vi "1500_DAQ.vi"(8 "error in":errorcluster) -> (0 "error out":errorcluster, 1 "输入":waveform(dbl)(graph), 2 "方波刺激":waveform(dbl)(graph), 3 "电阻值 2":dbl)   [LabVIEW 2016]
uses:
  <vilib>/DAQmx/write.llb/DAQmx Write (Analog Wfm 1Chan NSamp).vi
  <vilib>/DAQmx/read.llb/DAQmx Read (Analog Wfm 1Chan NSamp).vi
  <vilib>/Analysis/baseanly.llb/Mean (DBL).vi
  <vilib>/Waveform/WDTOps.llb/WDT Waveform Duration DBL.vi
  <vilib>/DAQmx/create/channels.llb/DAQmx Create Channel (AI-Voltage-Basic).vi
  <vilib>/DAQmx/configure/timing.llb/DAQmx Timing (Sample Clock).vi
  <vilib>/DAQmx/create/channels.llb/DAQmx Create Channel (AO-Voltage-Basic).vi
  <vilib>/DAQmx/miscellaneous.llb/DAQmx Fill In Error Info.vi
  <vilib>/measure/NI_MABase.lvlib
  <resource>/objmgr/daqmx.rc
  <vilib>/Analysis/NI_AALBase.lvlib
panel:
  out "阻值波形图表":dbl(graph)
  out "Resistance":dbl
  out "Negative Peak":dbl
  out "前半段波形图":dbl[](graph)
  out "后半段波形图 2":dbl[](graph)
  out "最小值":dbl
  out "mean":dbl caption="均值" format="%0.2f"
  in  "Holding Voltage":dbl
  in  "amplitude":dbl=0.02
  in  "Averaging":i32=7
  in  "frequency":dbl=20.0
  in  "下拉列表":u16(ring)=1 items=["Current Clamp", "Voltage Clamp"]
  out "Waveform Graph":waveform(dbl)[](graph)
  in  "Initialize?":bool
  out "实际采样率":dbl=1000.0 format="%0.2f"
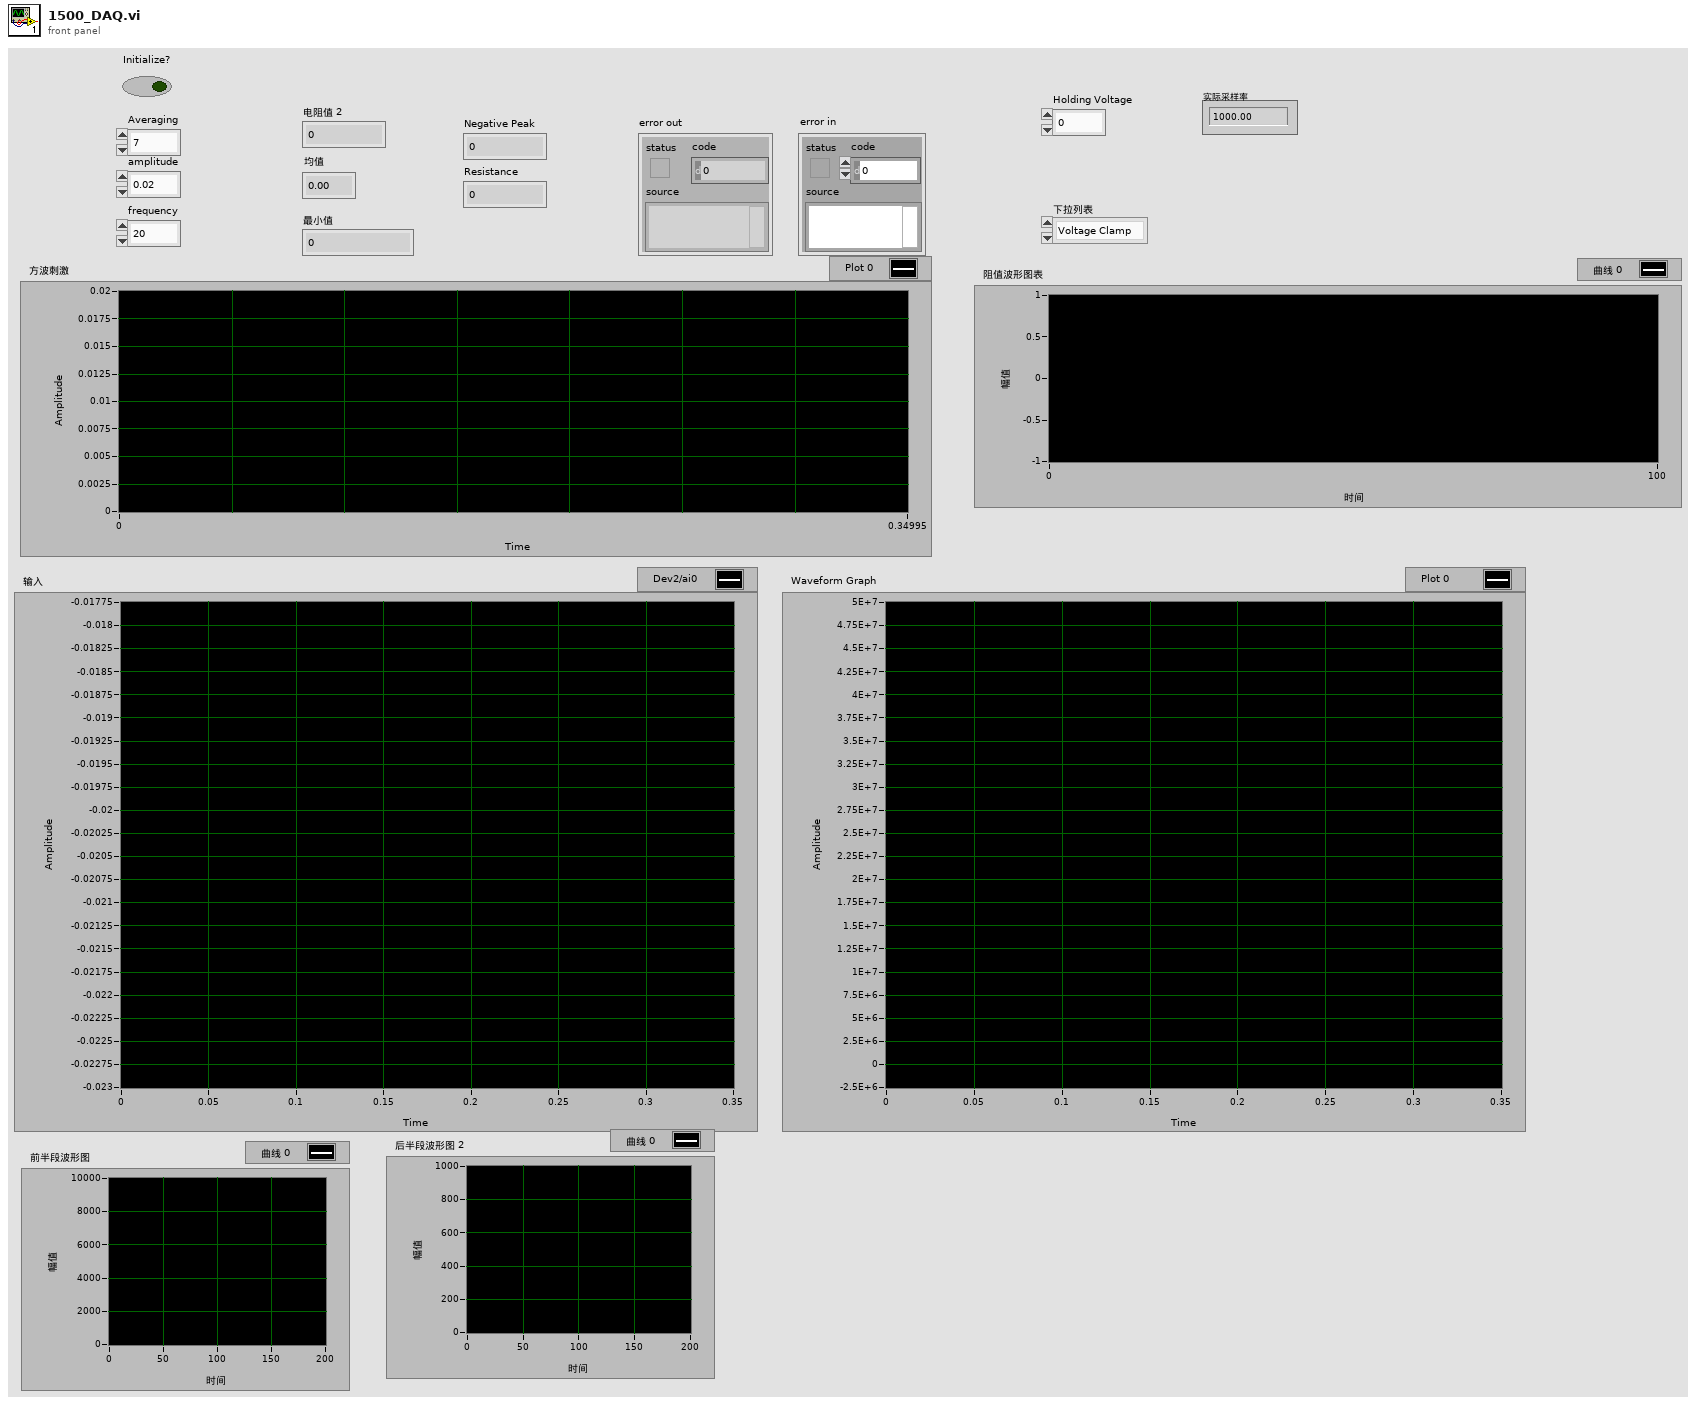
[diagram p1: front panel]
types:
  T1 = enum16{"Sine Wave", "Triangle Wave", "Square Wave", "Sawtooth Wave"}
  T2 = cluster{"Averaging":i32, "frequency":dbl, "amplitude":dbl, "Proportion":dbl, "Fs":dbl}
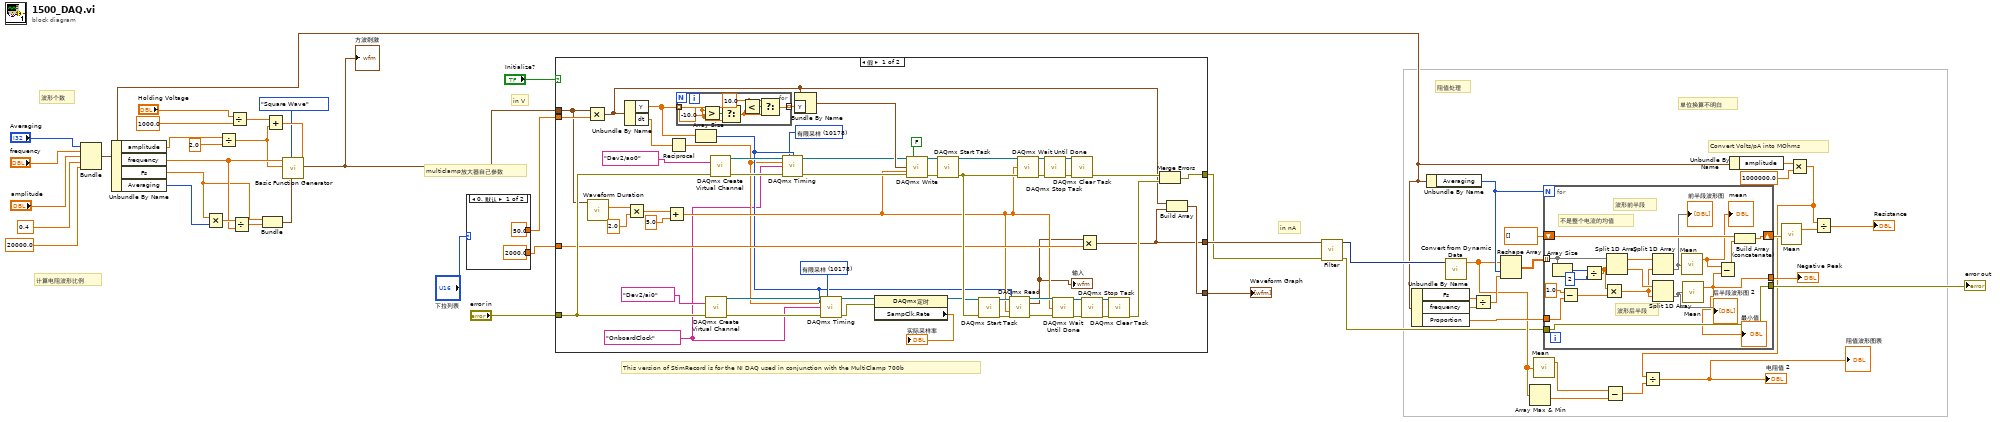
[diagram p0: block diagram]
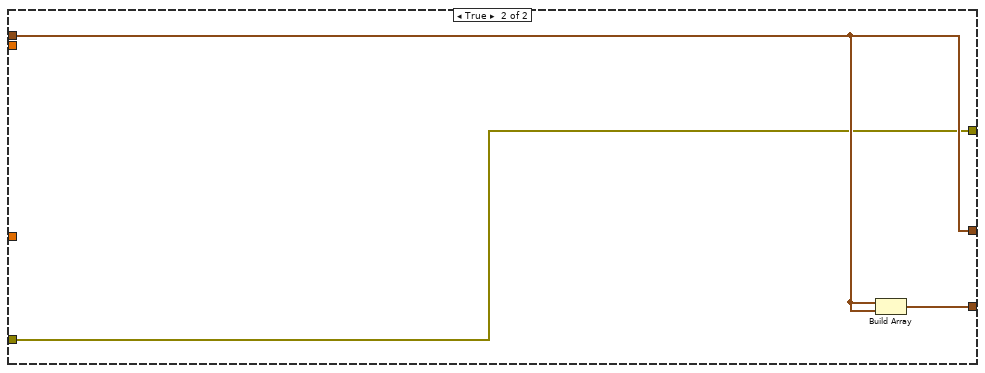
[diagram p2: hidden frame]
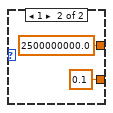
[diagram p3: hidden frame]
diagram:
  # "单位换算不明白"
  # "阻值处理"
  # "Convert Volts/pA into MOhms"
  # "波形个数"
  # "计算电阻波形比例"
  # "This version of StimRecord is for the NI DAQ used in conjunction with the MultiClamp 700b"
  # "multiclamp放大器自己参数"
  # "in V"
  # "in nA"
  n1 = Bundle("Averaging"="Averaging", "frequency"="frequency", "amplitude"="amplitude", "Proportion"=0.4, "Fs"=20000.0) -> (w1:T2)  [unwired: 1 in]
  n2 = Unbundle By Name(w1) -> ("amplitude"=w36:dbl, "frequency"=w37:dbl, "Fs"=w35:dbl, "Averaging"=w34:i32)
  n3 = Multiply(x=w35, y=w34) -> (x*y=w39:dbl)
  n4 = Divide(x=w36, y=2.0) -> (x/y=w31:dbl)
  n5 = Divide(x="Holding Voltage", y=1000.0) -> (x/y=w30:dbl)
  n6 = Divide(x=w39, y=w37) -> (x/y=w38:dbl)
  n7 = Bundle("Fs"=w35, w38) -> (w33:cluster{"Fs":dbl, dbl})  [unwired: 1 in]
  n8 = Add(x=w30, y=w31) -> (x+y=w32:dbl)
  n9 = call <vilib>:"Basic Function Generator.vi"("offset"=w32, "sampling info"=w33, "signal type"=T1."Square Wave", "amplitude"=w31, "frequency"=w37) -> ("signal out"=w26:waveform(dbl))  [unwired: 4 in, 2 out]
  "方波刺激" <- w26
  n10 = case shown="0, 默认" "下拉列表" {
    tunnel: [50.0 ("y") 2500000000.0 ("y")] -> w49
    tunnel: [2000.0 ("y") 0.1 ("y")] -> w48
    frame 0, Default {
    }
    frame 1 {
    }
  }
  n11 = case shown="假" "Initialize?" {
    tunnel: "error in" -> [w89 w117]
    tunnel: [w88 w117] -> w2
    tunnel: [w86 w119] -> w4
    tunnel: w26 -> [w75 w119]
    tunnel: [w87 w118] -> w50
    tunnel: w49 -> [w77 _]
    tunnel: w48 -> [w76 _]
    frame False {
      w57 = 10178 items=["有限采样"=10178, "连续采样"=10123, "硬件定时单点"=12522] ("sample mode")
      w56 = tag "OnboardClock" ("source")
      w66 = 10178 items=["有限采样"=10178, "连续采样"=10123, "硬件定时单点"=12522] ("sample mode")
      n12 = Multiply(x=w75, y=w77) -> (x*y=w84:waveform(dbl))
      n13 = call-poly <vilib>:"Waveform Duration.vi"("waveform in"=w75) -> ("duration"=w73:dbl)  [unwired: 8 in, 2 out]
      n14 = Unbundle By Name(w84) -> ("Y"=w79:dbl[], "dt"=w90:dbl)
      n15 = Multiply(x=w73, y=2.0) -> (x*y=w71:dbl)
      n16 = Add(x=w71, y=5.0) -> (x+y=w72:dbl)
      n17 = Reciprocal(x=w90) -> (1/x=w64:dbl)
      n18 = for {
        tunnel: [w116] -> w85 mode=indexing
        tunnel: w79 -> [w110] mode=indexing
        w111 = 10.0 ("t")
        w114 = -10.0 ("t")
        n19 = Greater?(x=w114, y=w110) -> (0:w115:bool)
        n20 = Select(t=w114, s=w115, f=w110) -> (s? t:f=w112:dbl)
        n21 = Less?(x=w111, y=w112) -> (x < y?=w113:bool)
        n22 = Select(t=w111, s=w113, f=w112) -> (s? t:f=w116:dbl)
      }
      n23 = Array Size(array=w79) -> (size(s)=w65:i32)
      n24 = call-poly <vilib>:"DAQmx Create Virtual Channel.vi"("physical channels"=tag "Dev2/ai0", "error in"=w89) -> ("task out"=w67:refnum<k21>, "error out"=w68:errorcluster)  [unwired: 12 in]
      n25 = call-poly <vilib>:"DAQmx Create Virtual Channel.vi"("physical channels"=tag "Dev2/ao0", "error in"=w89) -> ("task out"=w95:refnum<k21>, "error out"=w96:errorcluster)  [unwired: 12 in]
      n26 = call-poly <vilib>:"DAQmx Timing.vi"("task/channels in"=w95, "sample mode"=w57, "samples per channel"=w65, "rate"=w64, "source"=w56, "error in"=w96) -> ("task out"=w81:refnum<k21>, "error out"=w80:errorcluster)  [unwired: 8 in]
      n27 = Bundle By Name(cluster=w84, "Y"=w85) -> (w83:waveform(dbl))
      n28 = call-poly <vilib>:"DAQmx Timing.vi"("task/channels in"=w67, "sample mode"=w66, "samples per channel"=w65, "rate"=w64, "source"=w56, "error in"=w68) -> ("task out"=w62:refnum<k21>, "error out"=w61:errorcluster)  [unwired: 8 in]
      n29 = property class="DAQmx定时"(reference=w62, error in=w61) -> (reference out=w60:refnum<k21>, "SampClk.Rate"=→"实际采样率":dbl)  [unwired: 1 out]
      n30 = call-poly <vilib>:"DAQmx Write.vi"("task/channels in"=w81, "auto start"=FALSE, "data"=w83, "timeout"=w72, "error in"=w80) -> ("task out"=w91:refnum<k21>, "error out"=w82:errorcluster)  [unwired: 8 in, 1 out]
      n31 = call <vilib>:"DAQmx Start Task.vi"("task/channels in"=w91, "error in"=w82) -> ("task out"=w92:refnum<k21>, "error out"=w78:errorcluster)  [unwired: 12 in]
      n32 = call <vilib>:"DAQmx Start Task.vi"("task/channels in"=w60, "error in"=w78) -> ("task out"=w100:refnum<k21>, "error out"=w99:errorcluster)  [unwired: 12 in]
      n33 = call-poly <vilib>:"DAQmx Read.vi"("task/channels in"=w100, "number of samples per channel"=w65, "timeout"=w72, "error in"=w99) -> ("task out"=w106:refnum<k21>, "data"=w69:waveform(dbl), "error out"=w105:errorcluster)  [unwired: 9 in]
      "输入" <- w69
      n34 = call <vilib>:"DAQmx Wait Until Done.vi"("task/channels in"=w92, "timeout (sec)"=w72, "error in"=w78) -> ("task out"=w94:refnum<k21>, "error out"=w93:errorcluster)  [unwired: 11 in]
      n35 = call <vilib>:"DAQmx Stop Task.vi"("task/channels in"=w94, "error in"=w93) -> ("task out"=w97:refnum<k21>, "error out"=w98:errorcluster)  [unwired: 12 in]
      n36 = call <vilib>:"DAQmx Wait Until Done.vi"("task/channels in"=w106, "timeout (sec)"=w72, "error in"=w105) -> ("task out"=w104:refnum<k21>, "error out"=w103:errorcluster)  [unwired: 11 in]
      n37 = call <vilib>:"DAQmx Clear Task.vi"("task in"=w97, "error in"=w98) -> ("error out"=w108:errorcluster)  [unwired: 13 in]
      n38 = Multiply(x=w69, y=w76) -> (x*y=w86:waveform(dbl))
      n39 = call <vilib>:"DAQmx Stop Task.vi"("task/channels in"=w104, "error in"=w103) -> ("task out"=w102:refnum<k21>, "error out"=w101:errorcluster)  [unwired: 12 in]
      n40 = call <vilib>:"DAQmx Clear Task.vi"("task in"=w102, "error in"=w101) -> ("error out"=w107:errorcluster)  [unwired: 13 in]
      n41 = Merge Errors(w108, w107) -> (w88:errorcluster)
      n42 = Build Array(w84, w86) -> (w87:waveform(dbl)[])
    }
    frame True {
      n43 = Build Array(w119, w119) -> (w118:waveform(dbl)[])
    }
  }
  "Waveform Graph" <- w50
  n44 = call "Filter"("error in (no error)"=w2, "Signal"=w4) -> ("error out"=w3:errorcluster, "Filtered Signal"=w5:dynamicdata)  [unwired: 8 in]
  n45 = Unbundle By Name(w1) -> ("Fs"=w22:dbl, "frequency"=w21:dbl, "Proportion"=w13:dbl)
  n46 = Unbundle By Name(w1) -> ("Averaging"=w20:i32)
  n47 = call "Convert from Dynamic Data"("Dynamic Data Type"=w5) -> ("Array"=w9:dbl[])  [unwired: 3 in]
  n48 = Divide(x=w22, y=w21) -> (x/y=w25:dbl)
  n49 = Reshape Array(w9, w20, w25) -> (w24:dbl[][])
  n50 = Array Max & Min(array=w9) -> (min value=w8:dbl)  [unwired: 3 out]
  n51 = call-poly <vilib>:"Mean.vi"("X"=w9) -> ("mean"=w10:dbl)  [unwired: 1 out]
  n52 = for {
    N: w20 -> [_]
    tunnel: w24 -> [w128] mode=indexing
    tunnel: w3 -> [w135]
    shift-right: [w136] -> w23
    shift-left: dbl[] [] -> [w137]
    tunnel: [w121] -> w19
    tunnel: [w135] -> w16
    tunnel: w13 -> [w127]
    # "不是整个电流的均值"
    # "波形后半段"
    # "波形前半段"
    n53 = Array Size(array=w128) -> (size(s)=w125:i32)
    n54 = Subtract(x=1.0, y=w127) -> (x-y=w130:dbl)
    n55 = Divide(x=w125, y=2) -> (x/y=w132:dbl)
    n56 = Multiply(x=w132, y=w130) -> (x*y=w129:dbl)
    n57 = Split 1D Array(array=w128, index=w132) -> (first subarray=w124:dbl[], second subarray=w133:dbl[])
    n58 = Split 1D Array(array=w124, index=w129) -> (second subarray=w123:dbl[])  [unwired: 1 out]
    "前半段波形图" <- w123
    n59 = Split 1D Array(array=w133, index=w129) -> (second subarray=w122:dbl[])  [unwired: 1 out]
    "后半段波形图 2" <- w122
    n60 = call-poly <vilib>:"Mean.vi"("X"=w123) -> ("mean"=w120:dbl)  [unwired: 1 out]
    "mean" <- w120
    n61 = call-poly <vilib>:"Mean.vi"("X"=w122) -> ("mean"=w121:dbl)  [unwired: 1 out]
    "最小值" <- w121
    n62 = Subtract(x=w120, y=w121) -> (x-y=w126:dbl)
    n63 = Build Array (concatenate)(w137, w126) -> (w136:dbl[])
  }
  "Negative Peak" <- w19
  "error out" <- w16
  n64 = Subtract(x=w10, y=w8) -> (x-y=w7:dbl)
  n65 = Unbundle By Name(w1) -> ("amplitude"=w17:dbl)
  n66 = call-poly <vilib>:"Mean.vi"("X"=w23) -> ("mean"=w18:dbl)  [unwired: 1 out]
  n67 = Multiply(x=w17, y=1000000.0) -> (x*y=w11:dbl)
  n68 = Divide(x=w11, y=w7) -> (x/y=→"电阻值 2" →"阻值波形图表":dbl)
  n69 = Divide(x=w11, y=w18) -> (x/y=→"Resistance":dbl)
